vi "input_vel.vi"(2 "input":dbl, 3 "odrive":refnum<visa-resource-name>) -> (0 "error out":errorcluster, 1 "VISA resource name out":refnum<visa-resource-name>)   [LabVIEW 2018]
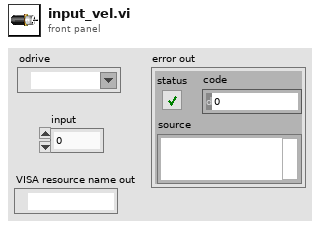
[diagram p1: front panel]
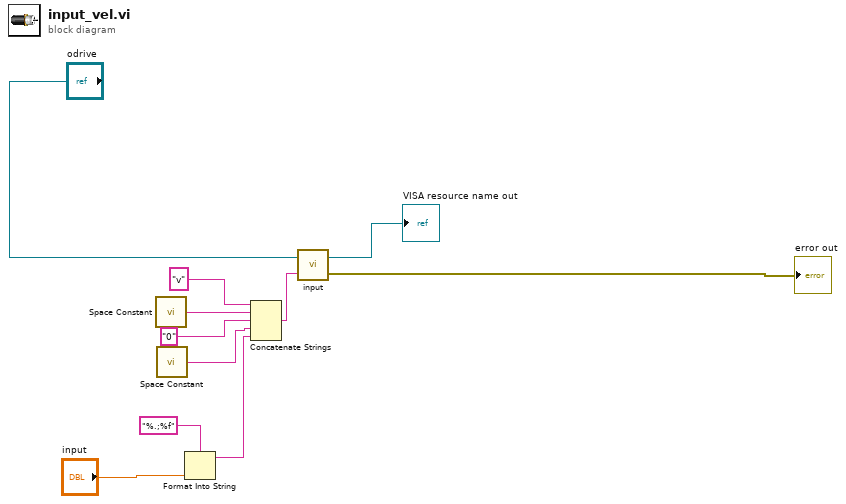
[diagram p0: block diagram]
diagram:
  n1 = call <vilib>:"Space Constant.vi"() -> ("String"=w9:string)
  n2 = call <vilib>:"Space Constant.vi"() -> ("String"=w11:string)
  n3 = Format Into String(format string="%.;%f", "input") -> (resulting string=w2:string)  [unwired: 2 in, 1 out]
  n4 = Concatenate Strings("v" ("write buffer"), w9, "0", w11, w2) -> (w7:string)
  n5 = call "input.vi"("commando"=w7, "VISA in"="odrive") -> ("error out"=→"error out":errorcluster, "VISA out"=→"VISA resource name out":refnum<visa-resource-name>)
